vi "Arduino___Lego_Mindstorms.vi"   [LabVIEW 2012]
uses:
  <vilib>/NXT/Block Support/NXT_InputPort.ctl
types:
  T1 = typedef "NXT_InputPort.ctl" = u8
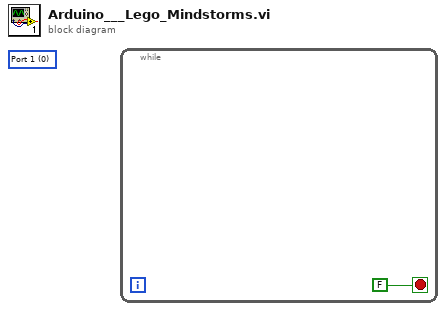
[diagram p0: block diagram]
diagram:
  (unwired) T1 0 items=["Port 1", "Port 2", "Port 3", "Port 4"] ("Input Port")
  n1 = while {
    stop <- FALSE stop-if-true
  }
